vi "Accekerometer Read values and Write to Serial.vi"(8 "error in (no error)":errorcluster) -> (0 "error out":errorcluster)   [LabVIEW 2014]
uses:
  <vilib>/LabVIEW Universal Transcriptor/LabVIEW to Arduino Transcriptor/Transcriptors/System API/Serial println string.vi
  <vilib>/LabVIEW Universal Transcriptor/Arduino MPU6050 Library/Arduino MPU6050.lvlib
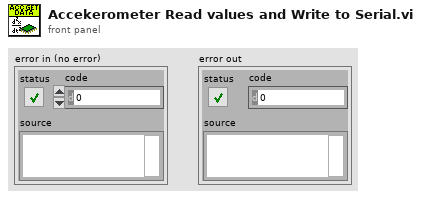
[diagram p1: front panel]
types:
  T1 = typedef "Arduino MPU6050.lvlib/MPU6050LibVector.ctl" = cluster{"XAxis":dbl, "YAxis":dbl, "ZAxis":dbl}
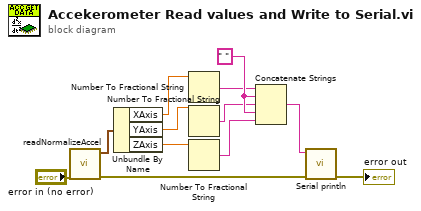
[diagram p0: block diagram]
diagram:
  w8 = " " ("F-format string")
  n1 = call <vilib>:"readNormalizeAccel.vi"("error in (no error)"="error in (no error)") -> ("error out"=w9:errorcluster, "Vector"=w10:T1)  [unwired: 9 in]
  n2 = Unbundle By Name(w10) -> ("XAxis"=w1:dbl, "YAxis"=w2:dbl, "ZAxis"=w3:dbl)
  n3 = Number To Fractional String(number=w1) -> (F-format string=w4:string)  [unwired: 3 in]
  n4 = Number To Fractional String(number=w2) -> (F-format string=w5:string)  [unwired: 3 in]
  n5 = Number To Fractional String(number=w3) -> (F-format string=w6:string)  [unwired: 3 in]
  n6 = Concatenate Strings(w4, w8, w5, w8, w6) -> (w7:string)
  n7 = call-poly <vilib>:"Serial println.vi"("Error In"=w9, "string in"=w7) -> ("Error Out"=→"error out":errorcluster)  [unwired: 9 in]
